vi "pause_bit_delete.vi"(1 "Массив с паузами":dbl[](array[numeric])) -> (0 "Массив без пауз":dbl[](array[numeric]))   [LabVIEW 2017]
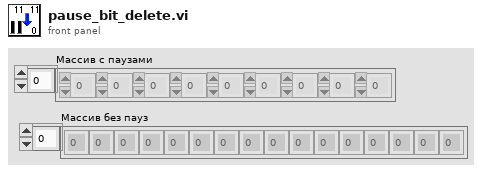
[diagram p1: front panel]
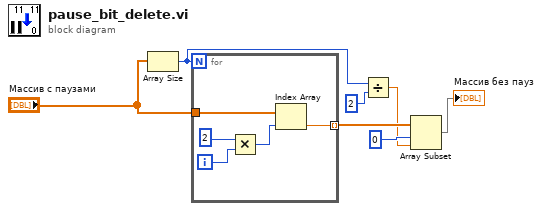
[diagram p0: block diagram]
diagram:
  n1 = Array Size(array="Массив с паузами") -> (size(s)=w5:i32)
  n2 = for {
    N: w5 -> [_]
    tunnel: "Массив с паузами" -> [w12]
    tunnel: [w9] -> w7 mode=indexing
    i -> [w10]
    n3 = Multiply(x=2, y=w10) -> (x*y=w8:i32)
    n4 = Index Array(array=w12, index=w8) -> (element=w9:dbl)
  }
  n5 = Divide(x=w5, y=2) -> (x/y=w3:dbl)
  n6 = Array Subset(array=w7, index=0, length=w3) -> (→"Массив без пауз":dbl[])
